vi "BioFeedback19(Adjustable View).vi"() -> ()   [LabVIEW 2016]
doc: "Use this template to build a producer/consumer design pattern. Use this template when you need to execute a process, such as data analysis, when a data source, such as a triggered acquisition, produces data at an uneven rate and you need to execute the process when the data becomes available."
uses:
  customSubVIs/8ChanWfmArray.ctl
  <vilib>/Utility/file.llb/Write Delimited Spreadsheet (string).vi
  <vilib>/Waveform/WDTFileIO.llb/Export Waveforms To Spreadsheet File (1D).vi
panel:
  out "Collecting Data":bool
  in  "Dismplay Min":dbl=10.0
  in  "Display Max":dbl=10.0
  in  "log filepath":path
  out "TrialStartTime":timestamp
  in  "Trial Duration":dbl=3.0
  out "Trial Number":dbl
  in  "Session Name":string="Test"
  out "loopTime":dbl=30.0 caption="Upper Cut-Off"
  in  "trial display data":path
  out "Disp Data":cluster{"queue out":refnum<queue>, dbl, dbl}[](array[cluster])
  in  "Target Percentage":dbl=10.0
  out "DisplayActivation":dbl
  out "DisplayBarActivation":dbl(slide) caption="Percent Activation" max=1.0 scale=0.0..100.0
  in  "Display Channel":dbl=0.5
  out "MVC Data":cluster{"queue out":refnum<queue>, dbl, dbl}[](array[cluster])
  out "Trial Name":string="Test"
  in  "Data Directory":path=path "C:/Users/Tinggroup/Desktop/VRMuscleActivationVisualizer/LabviewFiles/Data"
  out "GetMaxStartTime":timestamp
  in  "MVC Number":dbl=1.0
  in  "SecondsToAcquireMax":dbl=3.0
  in  "Frames Per Second":dbl=30.0 caption="Upper Cut-Off"
  in  "EMG Input Device\nProduct Type":string="USB-6009"
  out "raw data":dynamicdata(graph)
  out "dispSize":dbl=20.0 caption="Lower Cut-Off"
  out "mvcSize":dbl=300.0 caption="Upper Cut-Off"
  in  "MVC Window Size (s)":dbl=0.5
  in  "Display Window Size (s)":dbl=0.5
  in  "MVC Raw Path":path
  in  "trial raw data":path
  in  "trial filtered data":path
  in  "MVC Filtered Path":path
  in  "Sample rate (Hz)":dbl=1000.0 caption="Upper Cut-Off"
  out "fps":dbl=20.0 caption="Lower Cut-Off"
  out "rate":dbl=300.0 caption="Upper Cut-Off"
  in  "Set Parameters":bool
  out "lower":dbl=20.0 caption="Lower Cut-Off"
  out "upper":dbl=300.0 caption="Upper Cut-Off"
  in  "Lower Cut-Off":dbl=20.0
  in  "Upper Cut-Off":dbl=500.0
  in  "Mark":bool
  in  "End Trial":bool
  in  "Reset MVC":bool
  in  "Get MVC":bool
  in  "StartTrial":bool
  out "State":T1(ring)
  out "FilteredAndRectified":waveform(dbl)[](graph) caption="Filtered and Rectified"
  in  "stop":bool
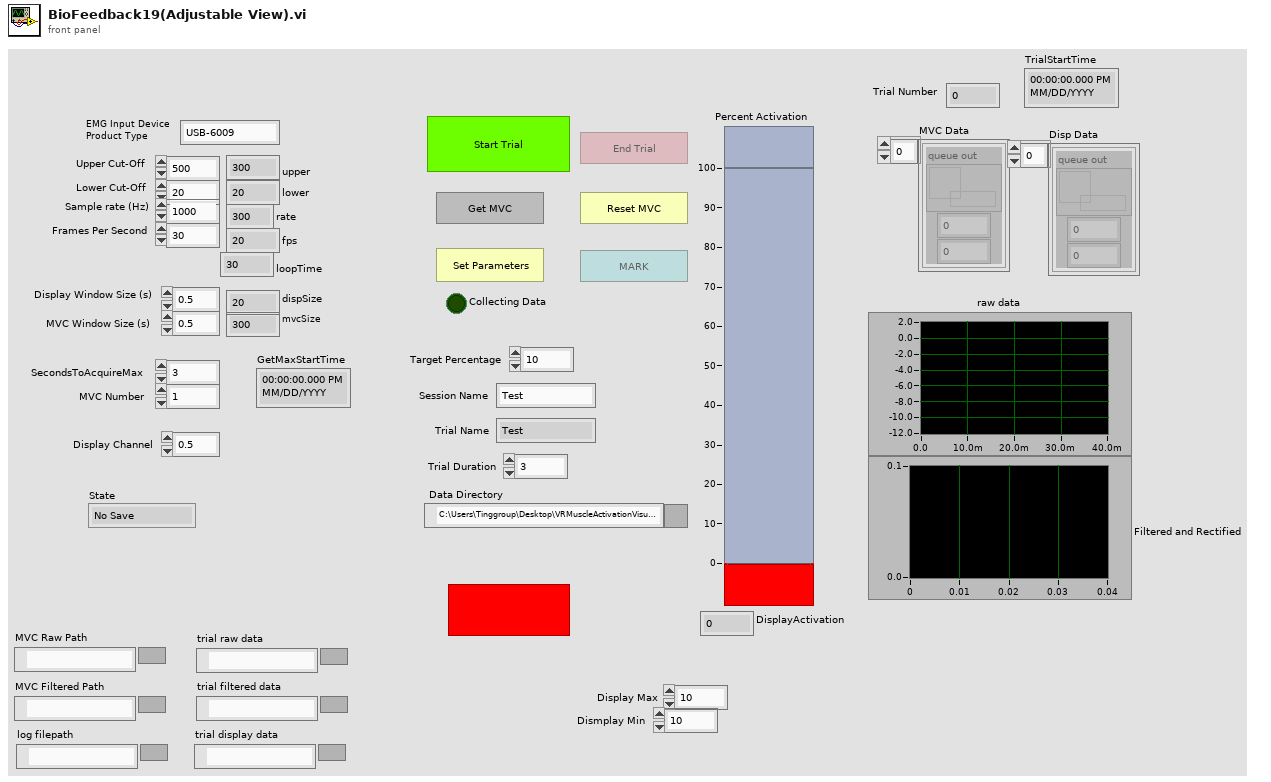
[diagram p1: front panel]
types:
  T1 = enum16{"No Save", "Acquiring Max", "Trial In Progress"}
  T2 = typedef "8ChanWfmArray.ctl" = waveform(dbl)[]
  T3 = enum8{"Enabled", "Disabled", "Disabled and Grayed Out"}
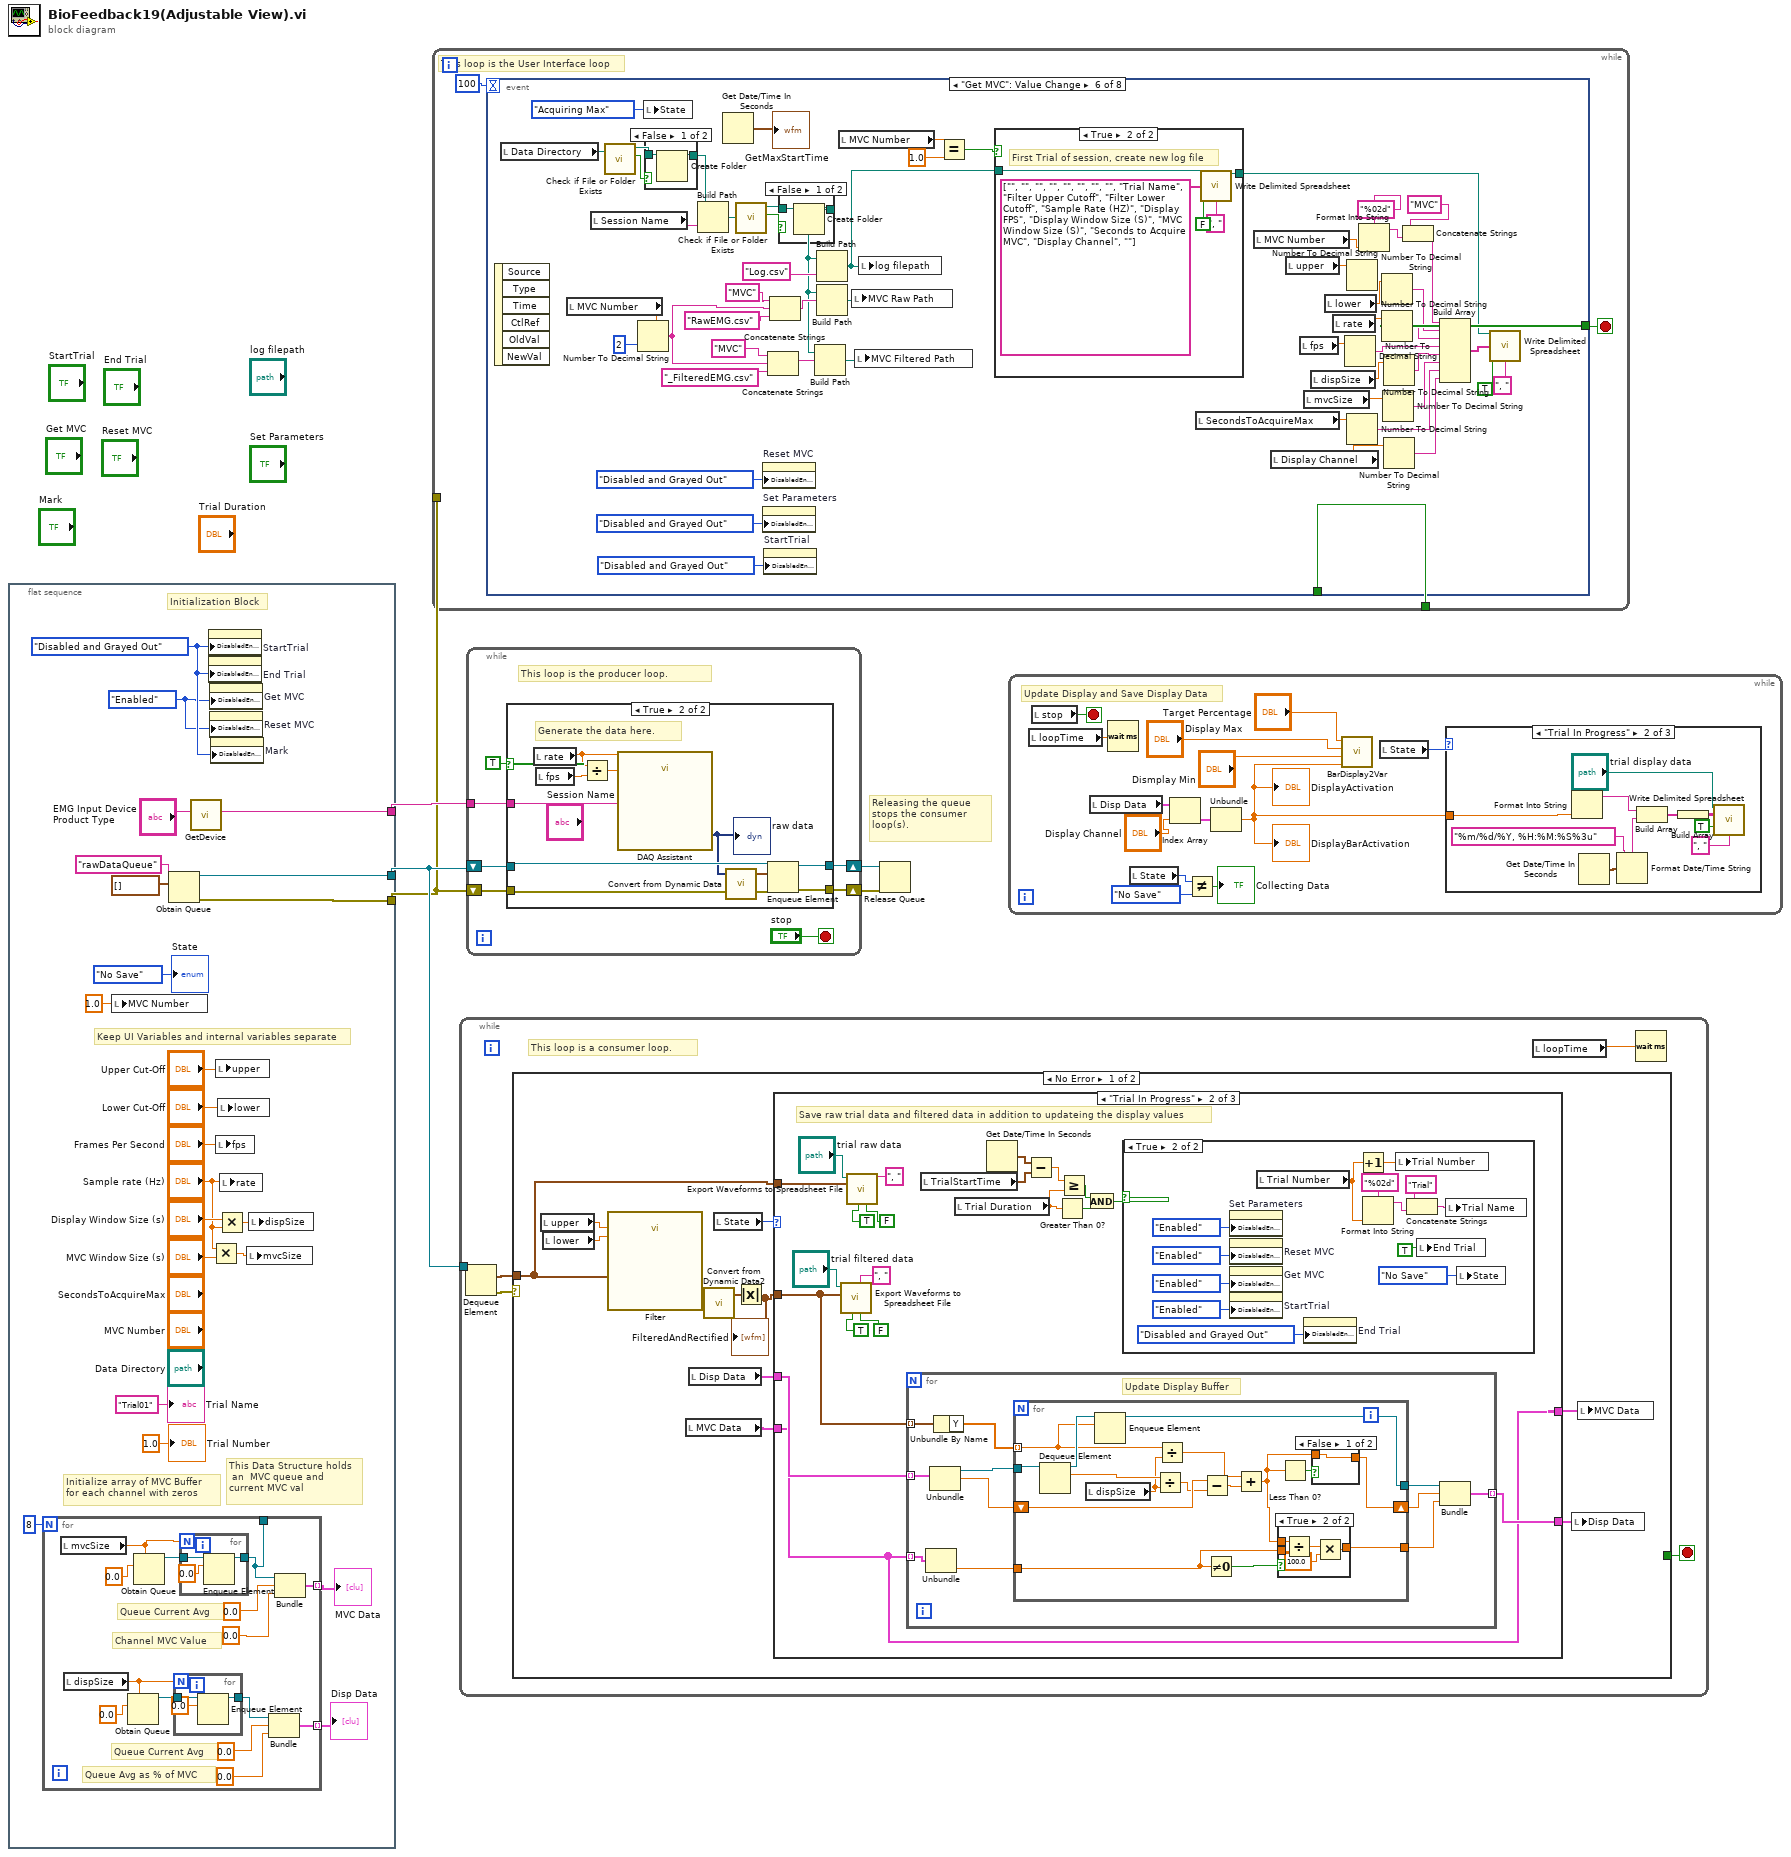
[diagram p0: block diagram]
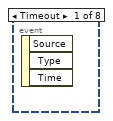
[diagram p4: hidden frame]
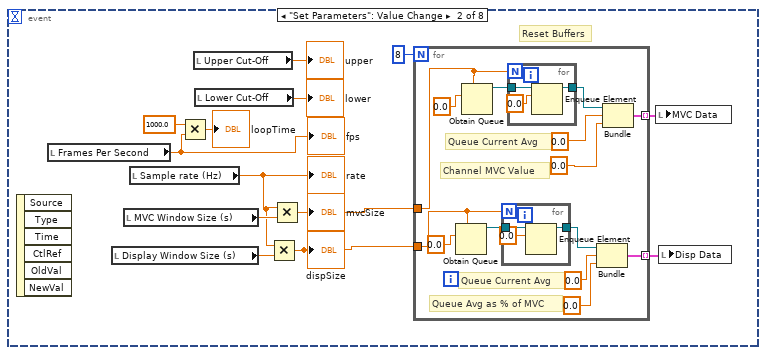
[diagram p5: hidden frame]
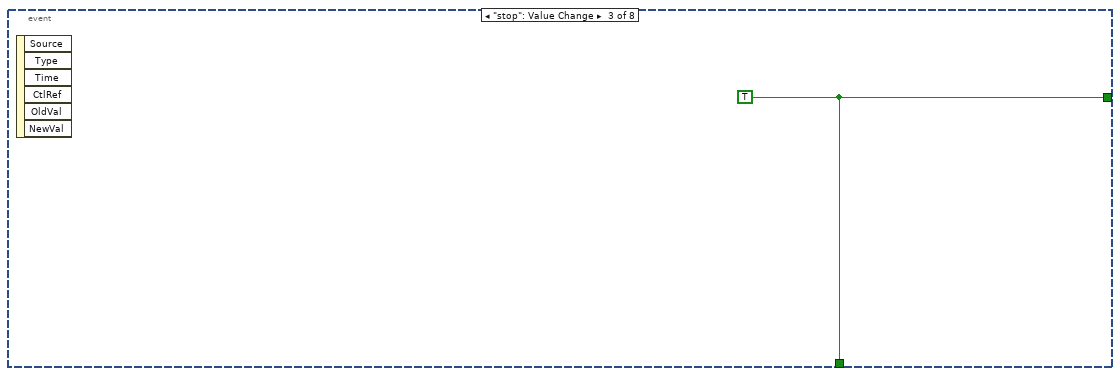
[diagram p6: hidden frame]
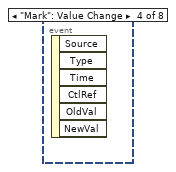
[diagram p7: hidden frame]
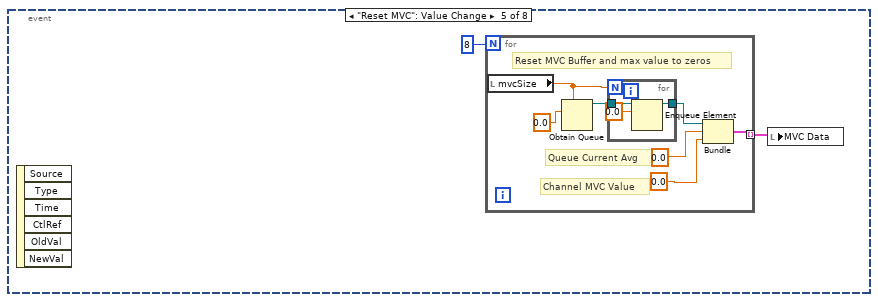
[diagram p8: hidden frame]
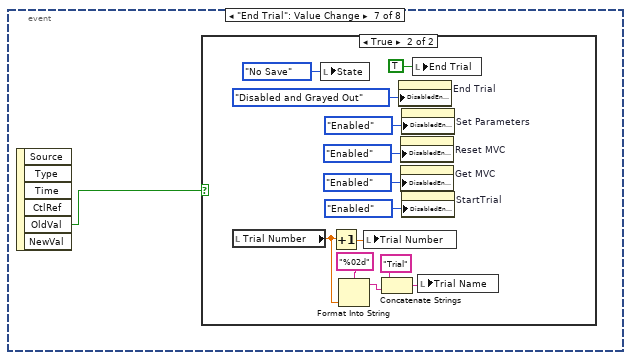
[diagram p12: hidden frame]
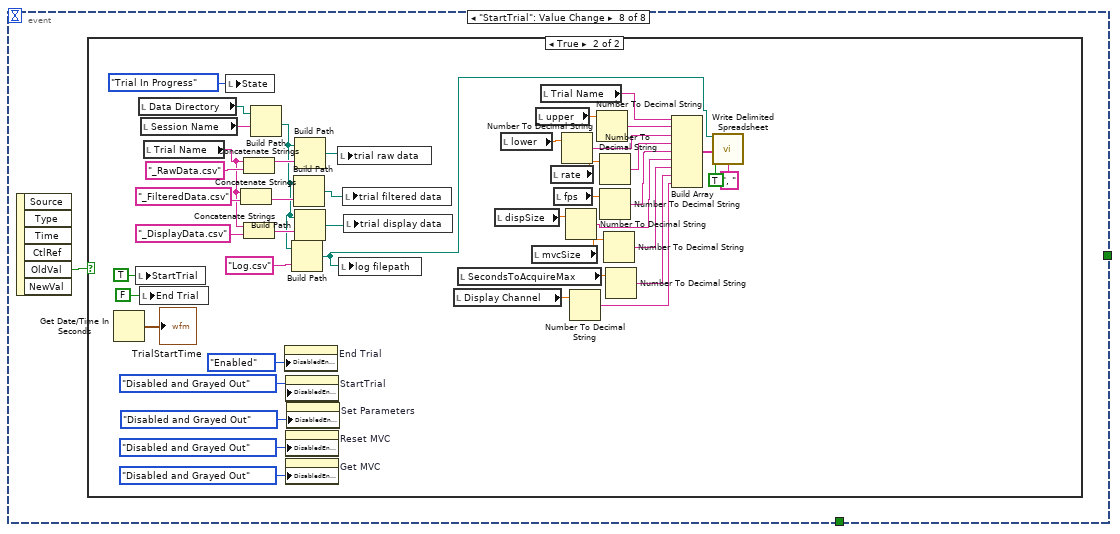
[diagram p14: hidden frame]
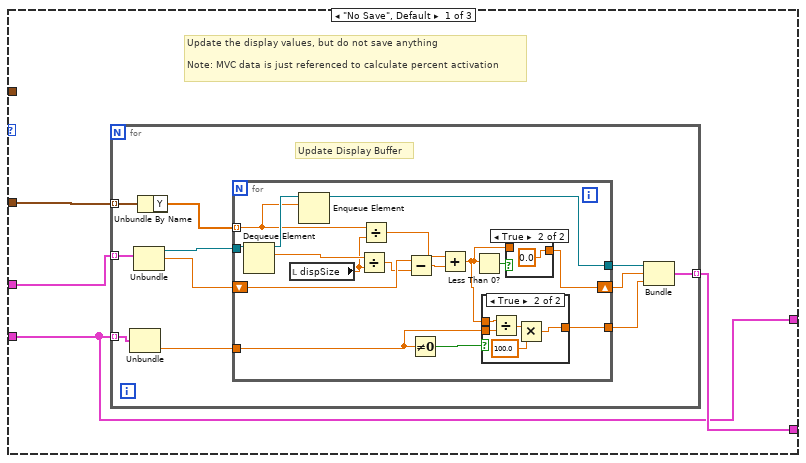
[diagram p16: hidden frame]
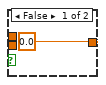
[diagram p18: hidden frame]
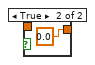
[diagram p20: hidden frame]
diagram:
  # "Releasing the queue stops the consumer loop(s)."
  n1 = flat-sequence {
    tunnel: [w19] -> w3
    tunnel: [w18] -> w2
    tunnel: [w21] -> w4
    frame #0 {
      w25 = T3."Enabled" ("Disabled")
      w26 = T3."Disabled and Grayed Out" ("Disabled")
      # "Keep UI Variables and internal variables separate"
      # "This Data Structure holds\n an  MVC queue and \ncurrent MVC val"
      # "Initialize array of MVC Buffer \nfor each channel with zeros"
      # "Initialization Block"
      n2 = for {
        N: 8 -> [_]
        tunnel: [w39] -> w11 mode=indexing
        tunnel: [w36] -> _
        tunnel: [w29] -> w10 mode=indexing
        # "Queue Avg as % of MVC"
        # "Queue Current Avg"
        # "Channel MVC Value"
        # "Queue Current Avg"
        n3 = local read "mvcSize"() -> (w40:dbl)
        n4 = local read "dispSize"() -> (w33:dbl)
        n5 = Obtain Queue(max queue size (-1, unlimited)=w33, element data type=0.0) -> (queue out=w30:refnum<queue>)  [unwired: 3 in, 2 out]
        n6 = Obtain Queue(max queue size (-1, unlimited)=w40, element data type=0.0) -> (queue out=w41:refnum<queue>)  [unwired: 3 in, 2 out]
        n7 = for {
          N: w33 -> [_]
          tunnel: w30 -> [w45]
          tunnel: [w43] -> w31
          n8 = Enqueue Element(queue=w45, element=0.0) -> (queue out=w43:refnum<queue>)  [unwired: 2 in, 2 out]
        }
        n9 = for {
          N: w40 -> [_]
          tunnel: w41 -> [w48]
          tunnel: [w46] -> w36
          n10 = Enqueue Element(queue=w48, element=0.0) -> (queue out=w46:refnum<queue>)  [unwired: 2 in, 2 out]
        }
        n11 = Bundle("queue out"=w31, 0.0, 0.0) -> (w29:cluster{"queue out":refnum<queue>, dbl, dbl})  [unwired: 1 in]
        n12 = Bundle("queue out"=w36, 0.0, 0.0) -> (w39:cluster{"queue out":refnum<queue>, dbl, dbl})  [unwired: 1 in]
      }
      "MVC Data" <- w11
      "Disp Data" <- w10
      n13 = local write "MVC Number"(1.0 ("MVC Number")) -> ()
      n14 = Obtain Queue(name (unnamed)="rawDataQueue", element data type=T2 [] ("initialized array")) -> (queue out=w19:refnum<queue>, error out=w18:errorcluster)  [unwired: 3 in, 1 out]
      n15 = call "GetDevice.vi"("EMG Input Device\nProduct Type"="EMG Input Device\nProduct Type") -> ("DAQmx Device Name"=w21:tag)  [unwired: 10 in]
      n16 = property on="StartTrial" class="Bool (strict)"("DisabledEnum"=w26) -> ()  [unwired: 2 in, 2 out]
      n17 = property on="End Trial" class="Bool (strict)"("DisabledEnum"=w26) -> ()  [unwired: 2 in, 2 out]
      n18 = property on="Get MVC" class="Bool"("DisabledEnum"=w25) -> ()  [unwired: 2 in, 2 out]
      n19 = property on="Reset MVC" class="Bool"("DisabledEnum"=w25) -> ()  [unwired: 2 in, 2 out]
      n20 = property on="Mark" class="Bool"("DisabledEnum"=w26) -> ()  [unwired: 2 in, 2 out]
      n21 = Multiply(x="Sample rate (Hz)", y="MVC Window Size (s)") -> (x*y=w13:dbl)
      n22 = local write "upper"("Upper Cut-Off") -> ()
      n23 = local write "fps"("Frames Per Second") -> ()
      n24 = Multiply(x="Display Window Size (s)", y="Sample rate (Hz)") -> (x*y=w16:dbl)
      n25 = local write "lower"("Lower Cut-Off") -> ()
      n26 = local write "rate"("Sample rate (Hz)") -> ()
      n27 = local write "mvcSize"(w13) -> ()
      n28 = local write "dispSize"(w16) -> ()
      "Trial Name" <- "Trial01" ("Trial Name")
      "State" <- T1."No Save" ("State")
      "Trial Number" <- 1.0 ("Trial Number")
    }
  }
  n29 = while {
    tunnel: [w51] -> _
    tunnel: w2 -> [_]
    stop <- w49 stop-if-true
    # "This loop is the User Interface loop"
    n30 = event shown="[5] \"Get MVC\": Value Change" {
      selector: _ -> [_ _ _ _ _ _ _ _]
      dyn-events: _ -> [_ _ _ _ _ _ _ _]
      timeout: u32 100 ("milliseconds to wait") -> [_ _ _ _ _ _ _ _]
      tunnel: [_ _ w85 _ _ _ _ _] -> w49
      tunnel: [_ _ w85 _ _ _ _ _] -> w51
      event Timeout {
        n31 = event-data() -> ()  [unwired: 1 in, 3 out]
      }
      event "Set Parameters": Value Change {
        # "Reset Buffers"
        n32 = event-data() -> ()  [unwired: 1 in, 6 out]
        n33 = local read "Frames Per Second"() -> (w52:dbl)
        "fps" <- w52
        n34 = local read "Display Window Size (s)"() -> (w62:dbl)
        n35 = local read "MVC Window Size (s)"() -> (w63:dbl)
        n36 = local read "Sample rate (Hz)"() -> (w60:dbl)
        "rate" <- w60
        n37 = Multiply(x=1000.0, y=w52) -> (x*y=→"loopTime":dbl)
        n38 = local read "Upper Cut-Off"() -> (→"upper":dbl)
        n39 = local read "Lower Cut-Off"() -> (→"lower":dbl)
        n40 = Multiply(x=w60, y=w62) -> (x*y=w58:dbl)
        "dispSize" <- w58
        n41 = Multiply(x=w60, y=w63) -> (x*y=w59:dbl)
        "mvcSize" <- w59
        n42 = for {
          N: 8 -> [_]
          tunnel: [w76] -> w56 mode=indexing
          tunnel: [w67] -> w57 mode=indexing
          tunnel: w59 -> [w66]
          tunnel: w58 -> [w65]
          # "Queue Avg as % of MVC"
          # "Queue Current Avg"
          # "Channel MVC Value"
          # "Queue Current Avg"
          n43 = Obtain Queue(max queue size (-1, unlimited)=w65, element data type=0.0) -> (queue out=w68:refnum<queue>)  [unwired: 3 in, 2 out]
          n44 = Obtain Queue(max queue size (-1, unlimited)=w66, element data type=0.0) -> (queue out=w77:refnum<queue>)  [unwired: 3 in, 2 out]
          n45 = for {
            N: w65 -> [_]
            tunnel: w68 -> [w81]
            tunnel: [w79] -> w69
            n46 = Enqueue Element(queue=w81, element=0.0) -> (queue out=w79:refnum<queue>)  [unwired: 2 in, 2 out]
          }
          n47 = for {
            N: w66 -> [_]
            tunnel: w77 -> [w84]
            tunnel: [w82] -> w73
            n48 = Enqueue Element(queue=w84, element=0.0) -> (queue out=w82:refnum<queue>)  [unwired: 2 in, 2 out]
          }
          n49 = Bundle("queue out"=w69, 0.0, 0.0) -> (w67:cluster{"queue out":refnum<queue>, dbl, dbl})  [unwired: 1 in]
          n50 = Bundle("queue out"=w73, 0.0, 0.0) -> (w76:cluster{"queue out":refnum<queue>, dbl, dbl})  [unwired: 1 in]
        }
        n51 = local write "MVC Data"(w56) -> ()
        n52 = local write "Disp Data"(w57) -> ()
      }
      event "stop": Value Change {
        w85 = TRUE
        n53 = event-data() -> ()  [unwired: 1 in, 6 out]
      }
      event "Mark": Value Change {
        n54 = event-data() -> ()  [unwired: 1 in, 6 out]
      }
      event "Reset MVC": Value Change {
        n55 = event-data() -> ()  [unwired: 1 in, 6 out]
        n56 = for {
          N: 8 -> [_]
          tunnel: [w88] -> w87 mode=indexing
          # "Channel MVC Value"
          # "Queue Current Avg"
          # "Reset MVC Buffer and max value to zeros"
          n57 = local read "mvcSize"() -> (w91:dbl)
          n58 = Obtain Queue(max queue size (-1, unlimited)=w91, element data type=0.0) -> (queue out=w90:refnum<queue>)  [unwired: 3 in, 2 out]
          n59 = for {
            N: w91 -> [_]
            tunnel: w90 -> [w97]
            tunnel: [w95] -> w92
            n60 = Enqueue Element(queue=w97, element=0.0) -> (queue out=w95:refnum<queue>)  [unwired: 2 in, 2 out]
          }
          n61 = Bundle("queue out"=w92, 0.0, 0.0) -> (w88:cluster{"queue out":refnum<queue>, dbl, dbl})  [unwired: 1 in]
        }
        n62 = local write "MVC Data"(w87) -> ()
      }
      event "Get MVC": Value Change {
        n63 = event-data() -> ()  [unwired: 1 in, 6 out]
        n64 = local read "Data Directory"() -> (w140:path)
        n65 = local read "MVC Number"() -> (w143:dbl)
        n66 = local read "Session Name"() -> (w142:string)
        n67 = call <vilib>:"Check if File or Folder Exists.vi"("path"=w140) -> ("file or folder exists?"=w137:bool, "dup path"=w144:path)  [unwired: 8 in, 1 out]
        n68 = Number To Decimal String(number=w143, width (-)=i16 2) -> (decimal integer string=w116:string)
        n69 = local write "State"(T1."Acquiring Max" ("State")) -> ()
        n70 = case shown="False" w137 {
          tunnel: w144 -> [w162 w163]
          tunnel: [w161 w163] -> w136
          frame False {
            n71 = Create Folder(path (use dialog)=w162) -> (created path=w161:path)  [unwired: 2 in, 2 out]
          }
          frame True {
          }
        }
        n72 = Build Path(base path=w136, name or relative path=w142) -> (appended path=w141:path)
        n73 = Get Date/Time In Seconds() -> (seconds since 1Jan1904=→"GetMaxStartTime":timestamp)
        n74 = call <vilib>:"Check if File or Folder Exists.vi"("path"=w141) -> ("file or folder exists?"=w139:bool, "dup path"=w138:path)  [unwired: 8 in, 1 out]
        n75 = property on="Reset MVC" class="Bool"("DisabledEnum"=T3."Disabled and Grayed Out" ("Disabled")) -> ()  [unwired: 2 in, 2 out]
        n76 = property on="Set Parameters" class="Bool"("DisabledEnum"=T3."Disabled and Grayed Out" ("Disabled")) -> ()  [unwired: 2 in, 2 out]
        n77 = property on="StartTrial" class="Bool (strict)"("DisabledEnum"=T3."Disabled and Grayed Out" ("Disabled")) -> ()  [unwired: 2 in, 2 out]
        n78 = Concatenate Strings("MVC" ("string"), w116, "_FilteredEMG.csv" ("string")) -> (w149:string)
        n79 = Concatenate Strings("MVC" ("string"), w116, "RawEMG.csv" ("string")) -> (w148:string)
        n80 = case shown="False" w139 {
          tunnel: w138 -> [w159 w160]
          tunnel: [w158 w160] -> w127
          frame False {
            n81 = Create Folder(path (use dialog)=w159) -> (created path=w158:path)  [unwired: 2 in, 2 out]
          }
          frame True {
          }
        }
        n82 = Build Path(base path=w127, name or relative path=w149) -> (appended path=w134:path)
        n83 = Build Path(base path=w127, name or relative path="Log.csv" ("string")) -> (appended path=w104:path)
        n84 = Build Path(base path=w127, name or relative path=w148) -> (appended path=w133:path)
        n85 = local read "MVC Number"() -> (w107:dbl)
        n86 = local write "MVC Raw Path"(w133) -> ()
        n87 = local write "MVC Filtered Path"(w134) -> ()
        n88 = local write "log filepath"(w104) -> ()
        n89 = Equal?(x=w107, y=1.0) -> (x = y?=w103:bool)
        n90 = case shown="True" w103 {
          tunnel: [w152 w154] -> w105
          tunnel: w104 -> [w152 w153]
          frame False {
            # "Do not create a new log file, use existing \nlog file"
          }
          frame True {
            # "First Trial of session, create new log file"
            n91 = call-poly <vilib>:"Write Delimited Spreadsheet.vi"("file path (dialog if empty)"=w153, "1D data"=string[] ["", "", "", "", "", "", "", "", "Trial Name", "Filter Upper Cutoff", "Filter Lower Cutoff", "Sample Rate (HZ)", "Display FPS", "Display Window Size (S)", "MVC Window Size (S)", "Seconds to Acquire MVC", "Display Channel", ""], "append to file? (new file:F)"=FALSE, "delimiter (\\t)"=", " ("delimiter (\\t)")) -> ("new file path (Not A Path if cancelled)"=w154:path)  [unwired: 10 in, 1 out]
          }
        }
        n92 = local read "SecondsToAcquireMax"() -> (w121:dbl)
        n93 = local read "MVC Number"() -> (w99:dbl)
        n94 = local read "Display Channel"() -> (w120:dbl)
        n95 = local read "upper"() -> (w126:dbl)
        n96 = local read "fps"() -> (w123:dbl)
        n97 = local read "mvcSize"() -> (w122:dbl)
        n98 = local read "dispSize"() -> (w117:dbl)
        n99 = local read "lower"() -> (w125:dbl)
        n100 = local read "rate"() -> (w124:dbl)
        n101 = Number To Decimal String(number=w123) -> (decimal integer string=w113:string)  [unwired: 1 in]
        n102 = Number To Decimal String(number=w126) -> ()  [unwired: 1 in, 1 out]
        n103 = Number To Decimal String(number=w121) -> (decimal integer string=w110:string)  [unwired: 1 in]
        n104 = Format Into String(format string="%02d", w99) -> (resulting string=w102:string)  [unwired: 2 in, 1 out]
        n105 = Number To Decimal String(number=w125) -> (decimal integer string=w115:string)  [unwired: 1 in]
        n106 = Number To Decimal String(number=w124) -> (decimal integer string=w114:string)  [unwired: 1 in]
        n107 = Number To Decimal String(number=w122) -> (decimal integer string=w111:string)  [unwired: 1 in]
        n108 = Number To Decimal String(number=w117) -> (decimal integer string=w112:string)  [unwired: 1 in]
        n109 = Number To Decimal String(number=w120) -> (decimal integer string=w109:string)  [unwired: 1 in]
        n110 = Concatenate Strings("MVC" ("string"), w102) -> (w98:string)
        n111 = Build Array(w98, w115, w114, w113, w112, w111, w110, w109) -> (w119:string[])
        n112 = call-poly <vilib>:"Write Delimited Spreadsheet.vi"("file path (dialog if empty)"=w105, "1D data"=w119, "append to file? (new file:F)"=TRUE, "delimiter (\\t)"=", " ("delimiter (\\t)")) -> ()  [unwired: 10 in, 2 out]
      }
      event "End Trial": Value Change {
        n113 = event-data() -> ("OldVal"=w164:bool)  [unwired: 1 in, 5 out]
        n114 = case shown="True" w164 {
          frame False {
          }
          frame True {
            n115 = local read "Trial Number"() -> (w169:dbl)
            n116 = local write "State"(T1."No Save" ("State")) -> ()
            n117 = Increment(x=w169) -> (x+1=w166:dbl)
            n118 = Format Into String(format string="%02d", w169) -> (resulting string=w168:string)  [unwired: 2 in, 1 out]
            n119 = local write "Trial Number"(w166) -> ()
            n120 = Concatenate Strings("Trial" ("string"), w168) -> (w170:string)
            n121 = property on="End Trial" class="Bool (strict)"("DisabledEnum"=T3."Disabled and Grayed Out" ("Disabled")) -> ()  [unwired: 2 in, 2 out]
            n122 = property on="Reset MVC" class="Bool"("DisabledEnum"=T3."Enabled" ("Disabled")) -> ()  [unwired: 2 in, 2 out]
            n123 = property on="Get MVC" class="Bool"("DisabledEnum"=T3."Enabled" ("Disabled")) -> ()  [unwired: 2 in, 2 out]
            n124 = property on="Set Parameters" class="Bool"("DisabledEnum"=T3."Enabled" ("Disabled")) -> ()  [unwired: 2 in, 2 out]
            n125 = property on="StartTrial" class="Bool (strict)"("DisabledEnum"=T3."Enabled" ("Disabled")) -> ()  [unwired: 2 in, 2 out]
            n126 = local write "End Trial"(TRUE ("End Trial")) -> ()
            n127 = local write "Trial Name"(w170) -> ()
          }
        }
      }
      event "StartTrial": Value Change {
        n128 = event-data() -> ("OldVal"=w178:bool)  [unwired: 1 in, 5 out]
        n129 = case shown="True" w178 {
          frame False {
          }
          frame True {
            n130 = Get Date/Time In Seconds() -> (seconds since 1Jan1904=→"TrialStartTime":timestamp)
            n131 = local write "StartTrial"(TRUE ("StartTrial")) -> ()
            n132 = local read "Data Directory"() -> (w214:path)
            n133 = local write "End Trial"(FALSE ("End Trial")) -> ()
            n134 = local read "Session Name"() -> (w213:string)
            n135 = local read "Trial Name"() -> (w196:string)
            n136 = local write "State"(T1."Trial In Progress" ("State")) -> ()
            n137 = Concatenate Strings(w196, "_FilteredData.csv" ("string")) -> (w218:string)
            n138 = Concatenate Strings(w196, "_RawData.csv" ("string")) -> (w216:string)
            n139 = Concatenate Strings(w196, "_DisplayData.csv" ("string")) -> (w220:string)
            n140 = Build Path(base path=w214, name or relative path=w213) -> (appended path=w195:path)
            n141 = property on="End Trial" class="Bool (strict)"("DisabledEnum"=T3."Enabled" ("Disabled")) -> ()  [unwired: 2 in, 2 out]
            n142 = property on="StartTrial" class="Bool (strict)"("DisabledEnum"=T3."Disabled and Grayed Out" ("Disabled")) -> ()  [unwired: 2 in, 2 out]
            n143 = property on="Reset MVC" class="Bool"("DisabledEnum"=T3."Disabled and Grayed Out" ("Disabled")) -> ()  [unwired: 2 in, 2 out]
            n144 = property on="Get MVC" class="Bool"("DisabledEnum"=T3."Disabled and Grayed Out" ("Disabled")) -> ()  [unwired: 2 in, 2 out]
            n145 = property on="Set Parameters" class="Bool"("DisabledEnum"=T3."Disabled and Grayed Out" ("Disabled")) -> ()  [unwired: 2 in, 2 out]
            n146 = Build Path(base path=w195, name or relative path="Log.csv" ("string")) -> (appended path=w179:path)
            n147 = Build Path(base path=w195, name or relative path=w218) -> (appended path=w212:path)
            n148 = Build Path(base path=w195, name or relative path=w216) -> (appended path=w211:path)
            n149 = Build Path(base path=w195, name or relative path=w220) -> (appended path=w221:path)
            n150 = local write "trial raw data"(w211) -> ()
            n151 = local write "log filepath"(w179) -> ()
            n152 = local write "trial filtered data"(w212) -> ()
            n153 = local write "trial display data"(w221) -> ()
            n154 = local read "Display Channel"() -> (w205:dbl)
            n155 = local read "SecondsToAcquireMax"() -> (w204:dbl)
            n156 = local read "dispSize"() -> (w202:dbl)
            n157 = local read "lower"() -> (w199:dbl)
            n158 = local read "mvcSize"() -> (w203:dbl)
            n159 = local read "upper"() -> (w198:dbl)
            n160 = local read "Trial Name"() -> (w192:string)
            n161 = local read "rate"() -> (w200:dbl)
            n162 = local read "fps"() -> (w201:dbl)
            n163 = Number To Decimal String(number=w199) -> (decimal integer string=w188:string)  [unwired: 1 in]
            n164 = Number To Decimal String(number=w202) -> (decimal integer string=w186:string)  [unwired: 1 in]
            n165 = Number To Decimal String(number=w205) -> (decimal integer string=w183:string)  [unwired: 1 in]
            n166 = Number To Decimal String(number=w198) -> (decimal integer string=w189:string)  [unwired: 1 in]
            n167 = Number To Decimal String(number=w200) -> (decimal integer string=w187:string)  [unwired: 1 in]
            n168 = Number To Decimal String(number=w201) -> (decimal integer string=w182:string)  [unwired: 1 in]
            n169 = Number To Decimal String(number=w203) -> (decimal integer string=w185:string)  [unwired: 1 in]
            n170 = Number To Decimal String(number=w204) -> (decimal integer string=w184:string)  [unwired: 1 in]
            n171 = Build Array(w192, w189, w188, w187, w182, w186, w185, w184, w183) -> (w181:string[])
            n172 = call-poly <vilib>:"Write Delimited Spreadsheet.vi"("file path (dialog if empty)"=w179, "1D data"=w181, "append to file? (new file:F)"=TRUE, "delimiter (\\t)"=", " ("delimiter (\\t)")) -> ()  [unwired: 10 in, 2 out]
          }
        }
      }
    }
  }
  n173 = while {
    tunnel: w3 -> [w224]
    stop <- w225 stop-if-true
    # "This loop is a consumer loop."
    n174 = Dequeue Element(queue=w224) -> (element=w226:T2, error out=w227:errorcluster)  [unwired: 2 in, 2 out]
    n175 = case shown="No Error" w227 {
      tunnel: w226 -> [w233 _]
      tunnel: [_ TRUE] -> w225
      frame No Error {
        n176 = local read "upper"() -> (w236:dbl)
        n177 = local read "lower"() -> (w235:dbl)
        n178 = call "Filter"("Lower Cut-Off"=w235, "Upper Cut-Off"=w236, "Signal"=w233) -> ("Filtered Signal"=w237:dynamicdata)  [unwired: 7 in, 1 out]
        n179 = local read "MVC Data"() -> (w231:cluster{"queue out":refnum<queue>, dbl, dbl}[])
        n180 = local read "Disp Data"() -> (w230:cluster{"queue out":refnum<queue>, dbl, dbl}[])
        n181 = call "Convert from Dynamic Data2"("Dynamic Data Type"=w237) -> ("Array of Waveform"=w238:waveform(dbl)[])  [unwired: 3 in]
        n182 = local read "State"() -> (w234:T1)
        n183 = Absolute Value(x=w238) -> (abs(x)=w232:waveform(dbl)[])
        "FilteredAndRectified" <- w232
        n184 = case shown="\"Trial In Progress\"" w234 {
          tunnel: w232 -> [w242 w289 w358]
          tunnel: w233 -> [_ w292 w359]
          tunnel: w231 -> [w239 w287 w349]
          tunnel: w230 -> [w241 w290 w348]
          tunnel: [w240 w288 w350] -> w228
          tunnel: [w239 w287 w351] -> w229
          frame "No Save", Default {
            # "Update the display values, but do not save anything\n\nNote: MVC data is just referenced to calculate percent activation"
            n185 = for {
              tunnel: w241 -> [w247] mode=indexing
              tunnel: w242 -> [w252] mode=indexing
              tunnel: [w248] -> w240 mode=indexing
              tunnel: w239 -> [w245] mode=indexing
              # "Update Display Buffer"
              n186 = Unbundle(w245) -> (w244:dbl)  [unwired: 2 out]
              n187 = Unbundle(w247) -> ("queue out"=w253:refnum<queue>, w246:dbl)  [unwired: 1 out]
              n188 = Unbundle By Name(w252) -> ("Y"=w251:dbl[])
              n189 = for {
                tunnel: w253 -> [w263]
                tunnel: w251 -> [w259] mode=indexing
                shift-right: [w256] -> w250
                shift-left: w246 -> [w268]
                tunnel: [w258] -> w249
                tunnel: w244 -> [w261]
                tunnel: [w257] -> w243
                n190 = Dequeue Element(queue=w263) -> (queue out=w260:refnum<queue>, element=w269:dbl)  [unwired: 2 in, 2 out]
                n191 = local read "dispSize"() -> (w266:dbl)
                n192 = Enqueue Element(queue=w260, element=w259) -> (queue out=w258:refnum<queue>)  [unwired: 2 in, 2 out]
                n193 = Divide(x=w269, y=w266) -> (x/y=w267:dbl)
                n194 = Divide(x=w259, y=w266) -> (x/y=w264:dbl)
                n195 = Subtract(x=w268, y=w267) -> (x-y=w265:dbl)
                n196 = Not Equal To 0?(x=w261) -> (x != 0?=w262:bool)
                n197 = Add(x=w264, y=w265) -> (x+y=w254:dbl)
                n198 = Less Than 0?(x=w254) -> (x < 0?=w255:bool)
                n199 = case shown="True" w262 {
                  tunnel: w261 -> [_ w277]
                  tunnel: [0.0 w273] -> w257
                  tunnel: w254 -> [_ w276]
                  frame False {
                  }
                  frame True {
                    n200 = Divide(x=w276, y=w277) -> (x/y=w274:dbl)
                    n201 = Multiply(x=w274, y=100.0) -> (x*y=w273:dbl)
                  }
                }
                n202 = case shown="True" w255 {
                  tunnel: [w270 0.0] -> w256
                  tunnel: w254 -> [w270 _]
                  frame False {
                  }
                  frame True {
                  }
                }
              }
              n203 = Bundle("queue out"=w249, w250, w243) -> (w248:cluster{"queue out":refnum<queue>, dbl, dbl})  [unwired: 1 in]
            }
          }
          frame "Trial In Progress" {
            # "Save raw trial data and filtered data in addition to updateing the display values"
            n204 = call-poly <vilib>:"Export Waveforms to Spreadsheet File.vi"("header? (write header:T)"=FALSE, "delimiter (Tab)"=", ", "append to file? (new file:F)"=TRUE, "waveforms"=w289, "file path (dialog if empty)"="trial filtered data") -> ()  [unwired: 5 in, 2 out]
            n205 = call-poly <vilib>:"Export Waveforms to Spreadsheet File.vi"("header? (write header:T)"=FALSE, "delimiter (Tab)"=", ", "append to file? (new file:F)"=TRUE, "waveforms"=w292, "file path (dialog if empty)"="trial raw data") -> ()  [unwired: 5 in, 2 out]
            n206 = for {
              tunnel: w290 -> [w315] mode=indexing
              tunnel: w289 -> [w320] mode=indexing
              tunnel: [w316] -> w288 mode=indexing
              tunnel: w287 -> [w313] mode=indexing
              # "Update Display Buffer"
              n207 = Unbundle(w313) -> (w312:dbl)  [unwired: 2 out]
              n208 = Unbundle(w315) -> ("queue out"=w321:refnum<queue>, w314:dbl)  [unwired: 1 out]
              n209 = Unbundle By Name(w320) -> ("Y"=w319:dbl[])
              n210 = for {
                tunnel: w321 -> [w331]
                tunnel: w319 -> [w327] mode=indexing
                shift-right: [w322] -> w318
                shift-left: w314 -> [w336]
                tunnel: [w326] -> w317
                tunnel: w312 -> [w329]
                tunnel: [w325] -> w311
                n211 = Dequeue Element(queue=w331) -> (queue out=w328:refnum<queue>, element=w337:dbl)  [unwired: 2 in, 2 out]
                n212 = local read "dispSize"() -> (w334:dbl)
                n213 = Enqueue Element(queue=w328, element=w327) -> (queue out=w326:refnum<queue>)  [unwired: 2 in, 2 out]
                n214 = Divide(x=w337, y=w334) -> (x/y=w335:dbl)
                n215 = Divide(x=w327, y=w334) -> (x/y=w332:dbl)
                n216 = Subtract(x=w336, y=w335) -> (x-y=w333:dbl)
                n217 = Not Equal To 0?(x=w329) -> (x != 0?=w330:bool)
                n218 = Add(x=w332, y=w333) -> (x+y=w323:dbl)
                n219 = case shown="True" w330 {
                  tunnel: w329 -> [_ w345]
                  tunnel: [0.0 w343] -> w325
                  tunnel: w323 -> [_ w344]
                  frame False {
                  }
                  frame True {
                    n220 = Divide(x=w344, y=w345) -> (x/y=w342:dbl)
                    n221 = Multiply(x=w342, y=100.0) -> (x*y=w343:dbl)
                  }
                }
                n222 = Less Than 0?(x=w323) -> (x < 0?=w324:bool)
                n223 = case shown="False" w324 {
                  tunnel: [w338 0.0] -> w322
                  tunnel: w323 -> [w338 _]
                  frame False {
                  }
                  frame True {
                  }
                }
              }
              n224 = Bundle("queue out"=w317, w318, w311) -> (w316:cluster{"queue out":refnum<queue>, dbl, dbl})  [unwired: 1 in]
            }
            n225 = local read "TrialStartTime"() -> (w283:timestamp)
            n226 = local read "Trial Duration"() -> (w279:dbl)
            n227 = Get Date/Time In Seconds() -> (seconds since 1Jan1904=w282:timestamp)
            n228 = Subtract(x=w282, y=w283) -> (x-y=w284:dbl)
            n229 = Greater Than 0?(x=w279) -> (x > 0?=w280:bool)
            n230 = Greater Or Equal?(x=w284, y=w279) -> (x >= y?=w278:bool)
            n231 = And(x=w278, y=w280) -> (x .and. y?=w281:bool)
            n232 = case shown="True" w281 {
              frame False {
              }
              frame True {
                n233 = property on="Set Parameters" class="Bool"("DisabledEnum"=T3."Enabled" ("Disabled")) -> ()  [unwired: 2 in, 2 out]
                n234 = property on="Reset MVC" class="Bool"("DisabledEnum"=T3."Enabled" ("Disabled")) -> ()  [unwired: 2 in, 2 out]
                n235 = property on="Get MVC" class="Bool"("DisabledEnum"=T3."Enabled" ("Disabled")) -> ()  [unwired: 2 in, 2 out]
                n236 = property on="StartTrial" class="Bool (strict)"("DisabledEnum"=T3."Enabled" ("Disabled")) -> ()  [unwired: 2 in, 2 out]
                n237 = local read "Trial Number"() -> (w304:dbl)
                n238 = property on="End Trial" class="Bool (strict)"("DisabledEnum"=T3."Disabled and Grayed Out" ("Disabled")) -> ()  [unwired: 2 in, 2 out]
                n239 = Increment(x=w304) -> (x+1=w310:dbl)
                n240 = Format Into String(format string="%02d", w304) -> (resulting string=w303:string)  [unwired: 2 in, 1 out]
                n241 = local write "Trial Number"(w310) -> ()
                n242 = Concatenate Strings("Trial" ("string"), w303) -> (w308:string)
                n243 = local write "End Trial"(TRUE ("End Trial")) -> ()
                n244 = local write "Trial Name"(w308) -> ()
                n245 = local write "State"(T1."No Save" ("State")) -> ()
              }
            }
          }
          frame "Acquiring Max" {
            # "Automatically Stop Listening for Max after Acquire Max Time is elapsed"
            n246 = call-poly <vilib>:"Export Waveforms to Spreadsheet File.vi"("header? (write header:T)"=FALSE, "delimiter (Tab)"=", ", "append to file? (new file:F)"=TRUE, "waveforms"=w358, "file path (dialog if empty)"="MVC Filtered Path") -> ()  [unwired: 5 in, 2 out]
            n247 = call-poly <vilib>:"Export Waveforms to Spreadsheet File.vi"("header? (write header:T)"=FALSE, "delimiter (Tab)"=", ", "append to file? (new file:F)"=TRUE, "waveforms"=w359, "file path (dialog if empty)"="MVC Raw Path") -> ()  [unwired: 5 in, 2 out]
            n248 = for {
              tunnel: w358 -> [w385] mode=indexing
              tunnel: w349 -> [w383] mode=indexing
              tunnel: [w377] -> w351 mode=indexing
              tunnel: w348 -> [w375] mode=indexing
              tunnel: [w369] -> w350 mode=indexing
              # "For each channel, update Moving Average for each channel"
              n249 = Unbundle(w383) -> ("queue out"=w376:refnum<queue>, w382:dbl, w381:dbl)
              n250 = Unbundle By Name(w385) -> ("Y"=w384:dbl[])
              n251 = Unbundle(w375) -> ("queue out"=w371:refnum<queue>, w374:dbl)  [unwired: 1 out]
              n252 = for {
                tunnel: w384 -> [w394] mode=indexing
                shift-right: [w399] -> w379
                shift-left: w382 -> [w411]
                shift-right: [w403] -> w380
                shift-left: w376 -> [w402]
                shift-right: [w405] -> w378
                shift-left: w381 -> [w404]
                tunnel: w374 -> [w392]
                shift-right: [w387] -> w372
                shift-left: _ -> [_]
                shift-right: [w396] -> w373
                shift-left: w371 -> [w389]
                # "Update Max if necessary"
                # "Update MVC queue current avg and \nmax value for each data point"
                n253 = Dequeue Element(queue=w389) -> (queue out=w398:refnum<queue>, element=w397:dbl)  [unwired: 2 in, 2 out]
                n254 = local read "dispSize"() -> (w395:dbl)
                n255 = Dequeue Element(queue=w402) -> (queue out=w401:refnum<queue>, element=w400:dbl)  [unwired: 2 in, 2 out]
                n256 = Enqueue Element(queue=w398, element=w394) -> (queue out=w396:refnum<queue>)  [unwired: 2 in, 2 out]
                n257 = local read "mvcSize"() -> (w409:dbl)
                n258 = Divide(x=w397, y=w395) -> (x/y=w393:dbl)
                n259 = Enqueue Element(queue=w401, element=w394) -> (queue out=w403:refnum<queue>)  [unwired: 2 in, 2 out]
                n260 = Divide(x=w394, y=w395) -> (x/y=w391:dbl)
                n261 = Subtract(x=w392, y=w393) -> (x-y=w390:dbl)
                n262 = Divide(x=w400, y=w409) -> (x/y=w410:dbl)
                n263 = Divide(x=w394, y=w409) -> (x/y=w407:dbl)
                n264 = Add(x=w391, y=w390) -> (x+y=w386:dbl)
                n265 = Subtract(x=w411, y=w410) -> (x-y=w408:dbl)
                n266 = Add(x=w407, y=w408) -> (x+y=w399:dbl)
                n267 = Less Than 0?(x=w386) -> (x < 0?=w388:bool)
                n268 = Greater?(x=w399, y=w404) -> (0:w406:bool)
                n269 = case shown="True" w388 {
                  tunnel: [w412 0.0] -> w387
                  tunnel: w386 -> [w412 _]
                  frame False {
                  }
                  frame True {
                  }
                }
                n270 = case shown="False" w406 {
                  tunnel: w399 -> [_ w415]
                  tunnel: [w414 w415] -> w405
                  tunnel: w404 -> [w414 _]
                  frame False {
                  }
                  frame True {
                  }
                }
              }
              n271 = Bundle("queue out"=w373, w372, 0.0) -> (w369:cluster{"queue out":refnum<queue>, dbl, dbl})  [unwired: 1 in]
              n272 = Bundle("queue out"=w380, w379, w378) -> (w377:cluster{"queue out":refnum<queue>, dbl, dbl})  [unwired: 1 in]
            }
            n273 = local read "GetMaxStartTime"() -> (w355:timestamp)
            n274 = local read "SecondsToAcquireMax"() -> (w353:dbl)
            n275 = Get Date/Time In Seconds() -> (seconds since 1Jan1904=w356:timestamp)
            n276 = Subtract(x=w356, y=w355) -> (x-y=w354:dbl)
            n277 = Greater Or Equal?(x=w354, y=w353) -> (x >= y?=w352:bool)
            n278 = case shown="True" w352 {
              frame False {
              }
              frame True {
                w365 = T3."Enabled" ("Disabled")
                n279 = local read "MVC Number"() -> (w368:dbl)
                n280 = property on="StartTrial" class="Bool (strict)"("DisabledEnum"=w365) -> ()  [unwired: 2 in, 2 out]
                n281 = property on="Reset MVC" class="Bool"("DisabledEnum"=w365) -> ()  [unwired: 2 in, 2 out]
                n282 = property on="Set Parameters" class="Bool"("DisabledEnum"=w365) -> ()  [unwired: 2 in, 2 out]
                n283 = Increment(x=w368) -> (x+1=w367:dbl)
                n284 = local write "MVC Number"(w367) -> ()
                n285 = local write "State"(T1."No Save" ("State")) -> ()
              }
            }
          }
        }
        n286 = local write "Disp Data"(w228) -> ()
        n287 = local write "MVC Data"(w229) -> ()
      }
      frame Error {
        # "Return true for any case which should stop the loop."
      }
    }
    n288 = local read "loopTime"() -> (w223:dbl)
    n289 = Wait (ms)(milliseconds to wait=w223) -> ()  [unwired: 1 out]
  }
  n290 = while {
    shift-right: [w419] -> w1
    shift-left: w2 -> [w420]
    shift-right: [w421] -> w5
    shift-left: w3 -> [w422]
    tunnel: w4 -> [w417]
    stop <- "stop" stop-if-true
    # "This loop is the producer loop."
    n291 = case shown="True" TRUE ("Case Constant\n(See Context Help)") {
      tunnel: w422 -> [w425 w435]
      tunnel: [w425 w434] -> w421
      tunnel: w420 -> [w424 w433]
      tunnel: [w424 w432] -> w419
      tunnel: w417 -> [_ w426]
      frame False {
      }
      frame True {
        # "Generate the data here."
        n292 = local read "rate"() -> (w429:dbl)
        n293 = local read "fps"() -> (w430:dbl)
        n294 = Divide(x=w429, y=w430) -> (x/y=w428:dbl)
        n295 = call "DAQ Assistant"("rate"=w429, "number of samples"=w428, "device name"=w426) -> ("data"=w427:dynamicdata)  [unwired: 13 in, 3 out]
        "raw data" <- w427
        n296 = call "Convert from Dynamic Data"("Dynamic Data Type"=w427) -> ("Array of Waveform"=w431:waveform(dbl)[])  [unwired: 3 in]
        n297 = Enqueue Element(queue=w435, element=w431, error in (no error)=w433) -> (queue out=w434:refnum<queue>, error out=w432:errorcluster)  [unwired: 1 in, 1 out]
      }
    }
  }
  n298 = Release Queue(queue=w5, error in (no error)=w1) -> ()  [unwired: 1 in, 3 out]
  n299 = while {
    stop <- w444 stop-if-true
    # "Update Display and Save Display Data"
    n300 = local read "loopTime"() -> (w441:dbl)
    n301 = local read "stop"() -> (w444:bool)
    n302 = local read "Disp Data"() -> (w447:cluster{"queue out":refnum<queue>, dbl, dbl}[])
    n303 = Wait (ms)(milliseconds to wait=w441) -> ()  [unwired: 1 out]
    n304 = local read "State"() -> (w437:T1)
    n305 = Index Array(array=w447, index="Display Channel") -> (element=w445:cluster{"queue out":refnum<queue>, dbl, dbl})
    n306 = Not Equal?(x=w437, y=T1."No Save" ("State")) -> (x != y?=→"Collecting Data":bool)
    n307 = Unbundle(w445) -> (w442:dbl)  [unwired: 2 out]
    "DisplayBarActivation" <- w442
    "DisplayActivation" <- w442
    n308 = call "BarDisplay2Var.vi"("Activation Percentage"=w442, "scale min"="Dismplay Min", "scale max"="Display Max", "Target Percentage"="Target Percentage") -> ()  [unwired: 8 in]
    n309 = local read "State"() -> (w443:T1)
    n310 = case shown="\"Trial In Progress\"" w443 {
      tunnel: w442 -> [_ w451 _]
      frame "No Save", Default {
      }
      frame "Trial In Progress" {
        n311 = Format Into String(w451) -> (resulting string=w454:string)  [unwired: 3 in, 1 out]
        n312 = Get Date/Time In Seconds() -> (seconds since 1Jan1904=w452:timestamp)
        n313 = Format Date/Time String(time format string (%c)="%m/%d/%Y, %H:%M:%S%3u", seconds (now)=w452) -> (date/time string=w453:string)  [unwired: 1 in]
        n314 = Build Array(w454, w453) -> (w455:string[])
        n315 = Build Array(w455) -> (w456:string[][])
        n316 = call-poly <vilib>:"Write Delimited Spreadsheet.vi"("file path (dialog if empty)"="trial display data", "2D data"=w456, "append to file? (new file:F)"=TRUE, "delimiter (\\t)"=", " ("delimiter (\\t)")) -> ()  [unwired: 10 in, 2 out]
      }
      frame "Acquiring Max" {
      }
    }
  }
